vi "ConfigUtilities - Update Mappings.vi"(6 "Channel Data in":T2 {"Dependent Node References" format="%.0x"}, 7 "Channel Path":string, 8 "error in (no error)":errorcluster, 9 "Channel Path Destinations":string[](array[string]), 10 "Channel Path Sources":string[](array[string]), 11 "Item Ref in":T1 format="%.0x") -> (0 "error out":errorcluster, 3 "Channel Data out":T2 {"Dependent Node References" format="%.0x"})   [LabVIEW 2016, in "UDP-Custom-Device System Explorer.lvlib"]
uses:
  UDP-Custom-Device System Explorer.lvlib
  <vilib>/NI Veristand/Custom Device API/Custom Device Item Ref.ctl
  <vilib>/NI VeriStand/Custom Device API/Custom Device API.lvlib
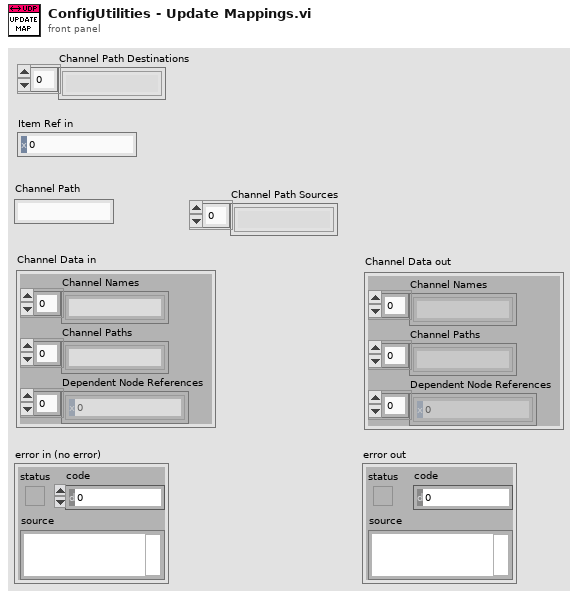
[diagram p1: front panel]
types:
  T1 = typedef "Custom Device API.lvlib/Custom Device Item Ref.ctl" = u64
  T2 = cluster{"Channel Names":string[], "Channel Paths":string[], "Dependent Node References":T1[]}
  T3 = typedef "Custom Device API.lvlib/Custom Device Item Info.ctl" = cluster{"Name":string, "Is Channel":bool, "GUID":string, "Is Waveform":bool}
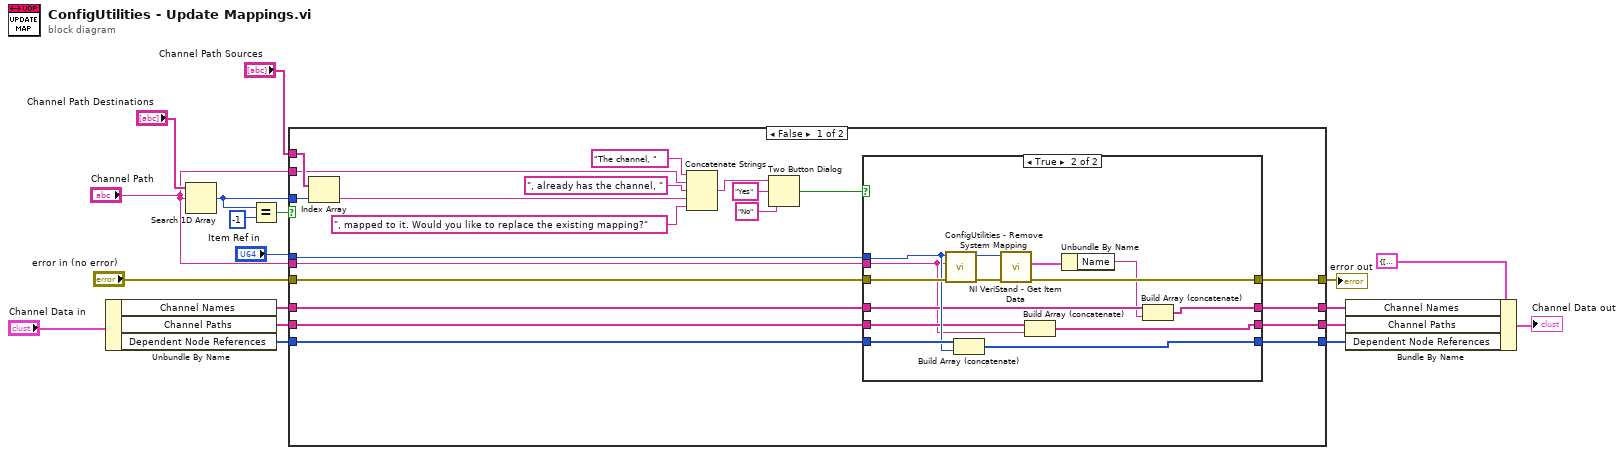
[diagram p0: block diagram]
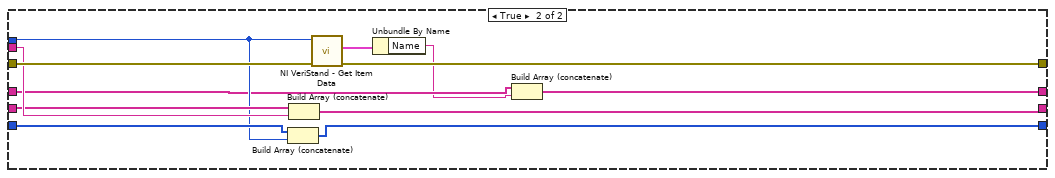
[diagram p3: hidden frame]
diagram:
  n1 = Unbundle By Name("Channel Data in") -> ("Channel Names"=w12:string[], "Channel Paths"=w11:string[], "Dependent Node References"=w10:T1[])
  n2 = Search 1D Array(1D array="Channel Path Destinations", element="Channel Path") -> (index of element=w14:i32)  [unwired: 1 in]
  n3 = Equal?(x=w14, y=-1) -> (x = y?=w16:bool)
  n4 = case shown="False" w16 {
    tunnel: "Channel Path Sources" -> [w39 _]
    tunnel: w14 -> [w38 _]
    tunnel: "Channel Path" -> [w35 _]
    tunnel: w12 -> [w29 w59]
    tunnel: w11 -> [w27 w64]
    tunnel: w10 -> [w26 w62]
    tunnel: "Item Ref in" -> [w25 w61]
    tunnel: "Channel Path" -> [w24 w65]
    tunnel: "error in (no error)" -> [w23 w68]
    tunnel: [w22 w66] -> w8
    tunnel: [w21 w63] -> w7
    tunnel: [w20 w60] -> w6
    tunnel: [w19 w67] -> w4
    frame False {
      n5 = Index Array(array=w39, index=w38) -> (element=w34:string)
      n6 = Concatenate Strings("The channel, " ("Path"), w35, ", already has the channel, " ("Path"), w34, ", mapped to it. Would you like to replace the existing mapping?" ("Path")) -> (w32:string)
      n7 = Two Button Dialog(message=w32, 1:"No" ("F button name (\"Cancel\")"), 2:"Yes" ("T button name (\"OK\")")) -> (T button?=w28:bool)
      n8 = case shown="True" w28 {
        tunnel: w29 -> [w43 w49]
        tunnel: w27 -> [w42 w46]
        tunnel: w26 -> [w41 w52]
        tunnel: w25 -> [_ w51]
        tunnel: w24 -> [_ w45]
        tunnel: w23 -> [w40 w57]
        tunnel: [w43 w47] -> w22
        tunnel: [w42 w44] -> w21
        tunnel: [w41 w50] -> w20
        tunnel: [w40 w53] -> w19
        frame False {
        }
        frame True {
          n9 = call "ConfigUtilities - Remove System Mapping.vi"("error in (no error)"=w57, "Channel Path Destination"=w45, "Item Ref in"=w51) -> ("error out"=w56:errorcluster, "Item Ref out"=w55:T1)  [unwired: 7 in]
          n10 = Build Array (concatenate)(w52, w51) -> (w50:T1[])
          n11 = call <vilib>:"NI VeriStand - Get Item Data.vi"("error in (no error)"=w56, "Item Ref in"=w55) -> ("error out"=w53:errorcluster, "Item Info"=w54:T3)  [unwired: 6 in, 2 out]
          n12 = Build Array (concatenate)(w46, w45) -> (w44:string[])
          n13 = Unbundle By Name(w54) -> ("Name"=w48:string)
          n14 = Build Array (concatenate)(w49, w48) -> (w47:string[])
        }
      }
    }
    frame True {
      n15 = Build Array (concatenate)(w62, w61) -> (w60:T1[])
      n16 = Build Array (concatenate)(w64, w65) -> (w63:string[])
      n17 = call <vilib>:"NI VeriStand - Get Item Data.vi"("error in (no error)"=w68, "Item Ref in"=w61) -> ("error out"=w67:errorcluster, "Item Info"=w69:T3)  [unwired: 6 in, 2 out]
      n18 = Unbundle By Name(w69) -> ("Name"=w58:string)
      n19 = Build Array (concatenate)(w59, w58) -> (w66:string[])
    }
  }
  "error out" <- w4
  n20 = Bundle By Name(cluster=T2 {"Channel Names"=[], "Channel Paths"=[], "Dependent Node References"=[]} ("Channel Data out"), "Channel Names"=w8, "Channel Paths"=w7, "Dependent Node References"=w6) -> (→"Channel Data out":T2)
